vi "Read Settings.vi"(8 "error in (no error)":errorcluster, 11 "KeithleyMeter in":refnum<class "KeithleyMeter.lvclass">) -> (0 "error out":errorcluster, 2 "Settings":string, 3 "KeithleyMeter out":refnum<class "KeithleyMeter.lvclass">)   [LabVIEW 2015, in "KeithleyMeter.lvclass"]
uses:
  KeithleyMeter.lvclass
  KeithleyMeter.lvclass/KeithleyMeter.ctl
  Instrument/Instrument.lvclass
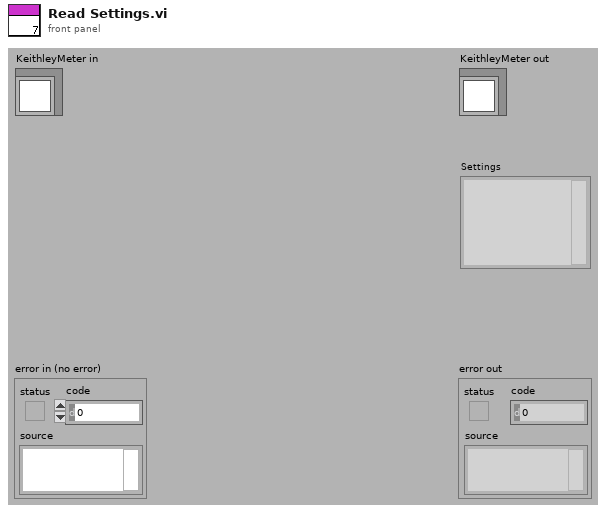
[diagram p1: front panel]
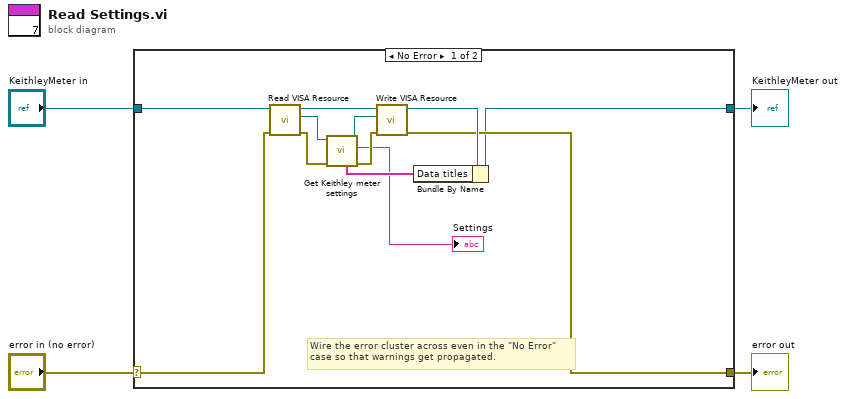
[diagram p0: block diagram]
diagram:
  n1 = case shown="No Error" "error in (no error)" {
    selector: "error in (no error)" -> [w12 w18]
    tunnel: [w9 w18] -> w3
    tunnel: [w7 w17] -> w1
    tunnel: "KeithleyMeter in" -> [w15 w17]
    frame No Error {
      # "Wire the error cluster across even in the \"No Error\"\ncase so that warnings get propagated."
      n2 = call "Read VISA Resource.vi"("error in (no error)"=w12, "Instrument.lvclass in"=w15) -> ("error out"=w11:errorcluster, "VISA Resource"=w13:refnum<visa-resource-name>, "Instrument.lvclass out"=w16:refnum<class "KeithleyMeter.lvclass">)  [unwired: 7 out]
      n3 = call "Get Keithley meter settings.vi"("error in (no error)"=w11, "VISA Resource Name"=w13) -> ("error out"=w10:errorcluster, "Parameters"=→"Settings":string, "VISA Resource Name Out"=w8:refnum<visa-resource-name>, "Data titles"=w6:string[])  [unwired: 1 in, 5 out]
      n4 = call "Write VISA Resource.vi"("error in (no error)"=w10, "VISA Resource"=w8, "Instrument.lvclass in"=w16) -> ("error out"=w9:errorcluster, "Instrument.lvclass out"=w14:refnum<class "KeithleyMeter.lvclass">)  [unwired: 7 out]
      n5 = Bundle By Name(cluster=w14, "Data titles"=w6) -> (w7:refnum<class "KeithleyMeter.lvclass">)
    }
    frame Error {
    }
  }
  "error out" <- w3
  "KeithleyMeter out" <- w1
